vi "Configure Instrument Prompt.vi"(8 "error in (no error)":errorcluster, 11 "Fluke Hydra 2625A in":refnum<class "Fluke Hydra 2625A.lvclass">) -> (0 "error out":errorcluster, 3 "Fluke Hydra 2625A out":refnum<class "Fluke Hydra 2625A.lvclass">)   [LabVIEW 2014, in "Generic Data Acquisition.lvlib" / "Fluke Hydra.lvlib" / "Fluke Hydra 2625A.lvclass"]
uses:
  Fluke Hydra 2625A.lvclass
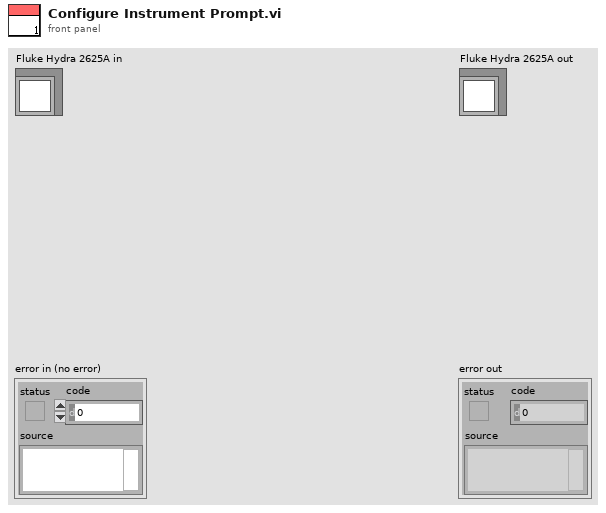
[diagram p1: front panel]
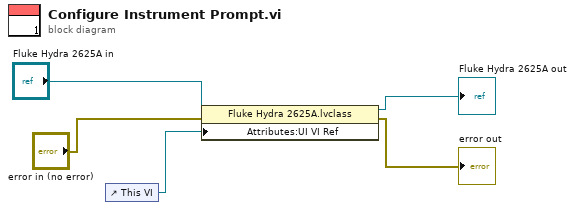
[diagram p0: block diagram]
diagram:
  n1 = control-ref of="This VI"() -> (w4:refnum<vi>)
  n2 = property class="Fluke Hydra 2625A.lvclass"(reference="Fluke Hydra 2625A in", error in="error in (no error)", "Attributes:UI VI Ref"=w4) -> (reference out=→"Fluke Hydra 2625A out":refnum<class "Fluke Hydra 2625A.lvclass">, error out=→"error out":errorcluster)
